vi "BncCore.vi"(8 "error in":errorcluster, 9 "queue error in":errorcluster, 10 "queue in":refnum<queue>, 11 "VISA resource":refnum<visa-resource-name>) -> (0 "error out":errorcluster, 2 "queue out":refnum<queue>)   [LabVIEW 2014]
uses:
  BNC_States.ctl
  SetSystemTypedef.ctl
  Command/Set C-Input.ctl
  Channel.ctl
  Command/Set C-Mode.ctl
  Command/Set C-Output.ctl
  Command/Set C-Enable.ctl
  <instrlib>/BNC/Public/Configure/Configure Sys (To) Mode (Single Shot).vi
  <instrlib>/BNC/Public/Configure/Configure Sys (To) Mode (Normal).vi
  <instrlib>/BNC/Public/Configure/Configure Sys (To) Mode (Duty Cycle).vi
  <instrlib>/BNC/Public/Configure/Configure Sys (To) Mode (Burst).vi
  <instrlib>/BNC/Public/Configure/Configure Chan Mode (Normal).vi
  <instrlib>/BNC/Berkeley Nucleonics 500 Series.lvlib
  <userlib>/Utility/ErrorLog_lib.lvlib
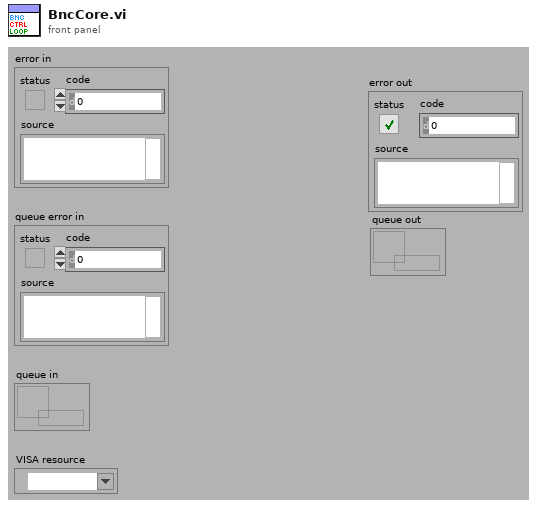
[diagram p1: front panel]
types:
  T1 = typedef "SetSystemTypedef.ctl" = cluster{"Mode":enum16{"Normal", "Single Shot", "Duty Cycle", "Burst"}, "Sys Ext Mode":enum16{"Disabled", "Triggered", "Gated", "Triggered & Gated"}, "Rep.Rate":dbl, "Burst#":i32}
  T2 = enum16{"Disabled", "Pulse Inhibit", "Output Inhibit", "Channel"}
  T3 = typedef "Set C-Input.ctl" = cluster{"Channel":T4, "Sync Source":T4}
  T4 = typedef "Channel.ctl" = i32
  T5 = typedef "Set C-Mode.ctl" = cluster{"Channel":T4, "Delay":dbl, "Width":dbl}
  T6 = typedef "Set C-Output.ctl" = cluster{"Channel":T4, "Polarity":bool}
  T7 = typedef "Set C-Enable.ctl" = cluster{"Channel":T4, "Enable":bool}
  T8 = typedef "BNC_States.ctl" = cluster{"State":enum16{"Initialize", "Set System", "Set C-Input", "Set C-Mode", "Set C-Output", "Set C-Enable", "Manl_Trig", "Run", "Stop", "Query C Number", "Query Status", "Close", "Quit"}, "Para.":variant}
  T9 = enum16{"Initialize", "Set System", "Set C-Input", "Set C-Mode", "Set C-Output", "Set C-Enable", "Manl_Trig", "Run", "Stop", "Query C Number", "Query Status", "Close", "Quit"}
  T10 = enum16{"Normal", "Single Shot", "Duty Cycle", "Burst"}
  T11 = enum16{"Disabled", "Triggered", "Gated", "Triggered & Gated"}
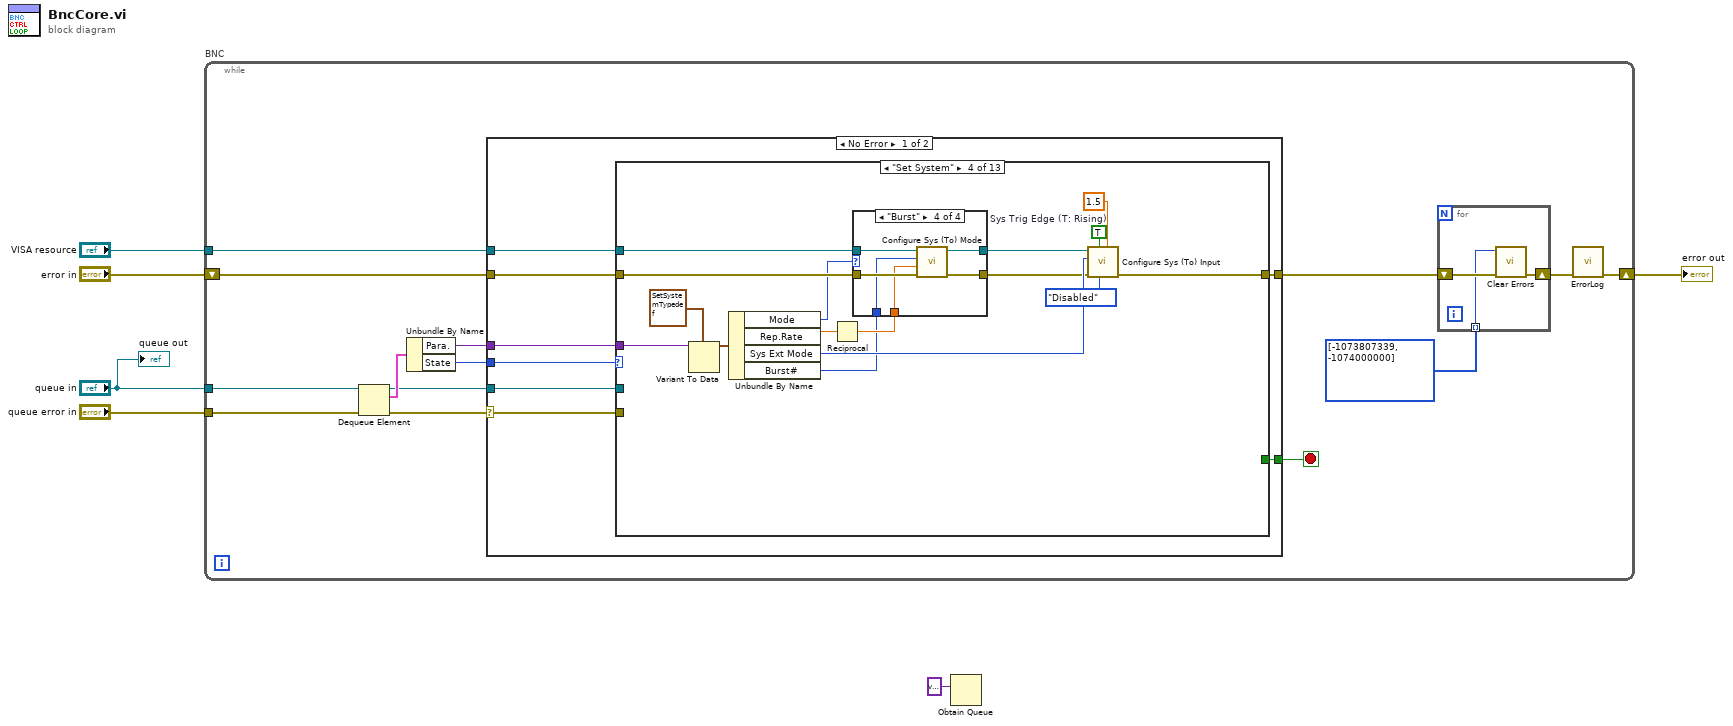
[diagram p0: block diagram]
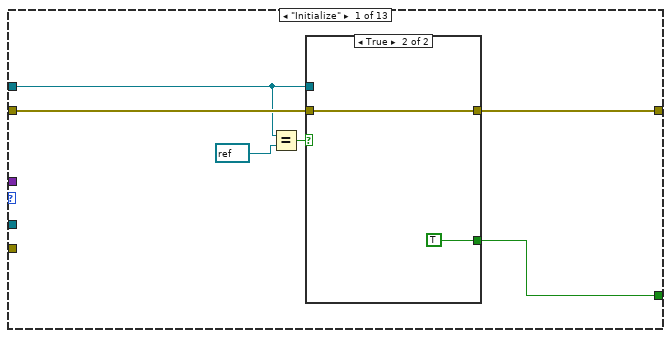
[diagram p2: hidden frame]
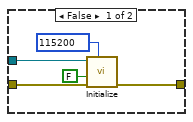
[diagram p3: hidden frame]
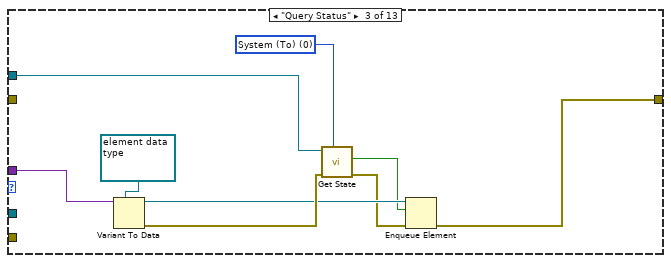
[diagram p5: hidden frame]
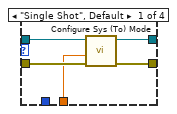
[diagram p6: hidden frame]
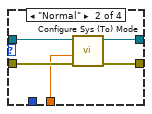
[diagram p7: hidden frame]
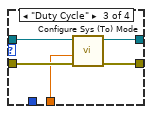
[diagram p8: hidden frame]
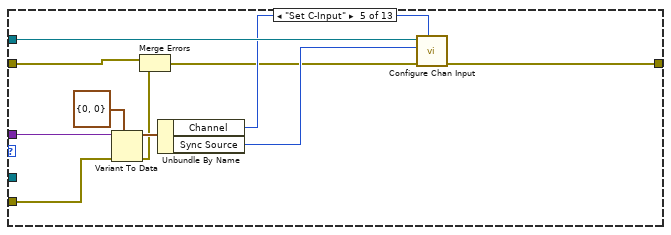
[diagram p9: hidden frame]
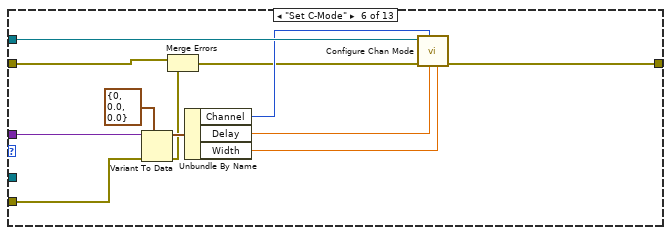
[diagram p10: hidden frame]
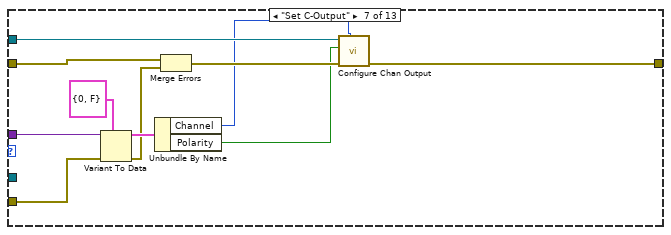
[diagram p11: hidden frame]
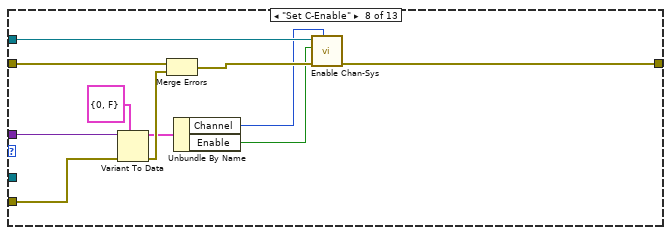
[diagram p12: hidden frame]
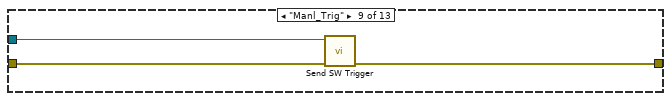
[diagram p13: hidden frame]
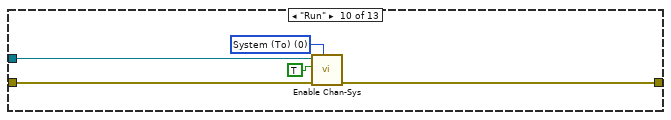
[diagram p14: hidden frame]
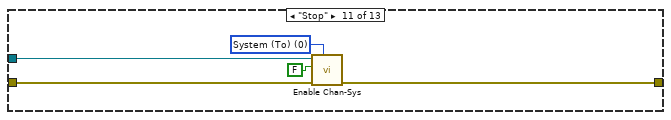
[diagram p15: hidden frame]
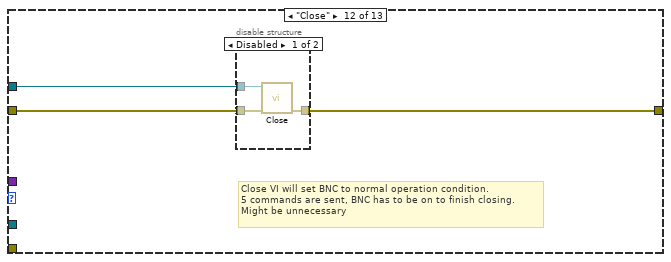
[diagram p16: hidden frame]
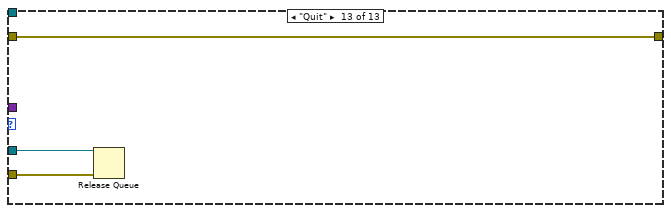
[diagram p18: hidden frame]
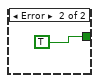
[diagram p19: hidden frame]
diagram:
  n1 = while "BNC" {
    tunnel: "queue in" -> [w20]
    tunnel: "VISA resource" -> [w15]
    shift-right: [w7] -> w2
    shift-left: "error in" -> [w10]
    tunnel: "queue error in" -> [w11]
    stop <- w12 stop-if-true
    n2 = Dequeue Element(queue=w20, error in (no error)=w11) -> (queue out=w16:refnum<queue>, element=w19:T8, error out=w13:errorcluster)  [unwired: 1 in, 1 out]
    n3 = Unbundle By Name(w19) -> ("Para."=w17:variant, "State"=w18:T9)
    n4 = case shown="No Error" w13 {
      selector: w13 -> [w26 _]
      tunnel: w18 -> [w31 _]
      tunnel: w17 -> [w30 _]
      tunnel: w16 -> [w29 _]
      tunnel: w15 -> [w28 _]
      tunnel: w10 -> [w27 _]
      tunnel: [w25 _] -> w14
      tunnel: [w24 TRUE] -> w12
      frame No Error {
        n5 = case shown="\"Set System\"" w31 {
          tunnel: w26 -> [_ _ _ _ w99 w110 w120 w131 _ _ _ _ w158]
          tunnel: w30 -> [_ _ w51 w65 w100 w113 w121 w133 _ _ _ _ _]
          tunnel: w29 -> [_ _ _ _ _ _ _ _ _ _ _ _ w159]
          tunnel: w28 -> [w33 _ w54 w69 w101 w114 w125 w135 w137 w142 w147 w151 _]
          tunnel: w27 -> [w37 w45 _ w70 w92 w103 w117 w136 w139 w143 w148 w152 w157]
          tunnel: [w36 w45 w47 w68 w102 w112 w124 w134 w138 w141 w146 w150 w157] -> w25
          tunnel: [w32 _ _ _ _ _ _ _ _ _ _ _ _] -> w24
          frame "Initialize" {
            n6 = Equal?(x=w33, y=refnum<visa-resource-name> refnum ("VISA resource")) -> (x = y?=w35:bool)
            n7 = case shown="True" w35 {
              tunnel: w33 -> [w42 _]
              tunnel: w37 -> [w41 w44]
              tunnel: [w40 w44] -> w36
              tunnel: [_ TRUE] -> w32
              frame False {
                w38 = u32 115200 items=["4800"=4600, "9600"=9600, "19200"=19200, "38400"=38400, "57600"=57600, "115200"=115200] ("Baud Rate (115200)")
                n8 = call <instrlib>:"Initialize.vi"("Baud Rate (115200)"=w38, "error in (no error)"=w41, "Reset? (T: Yes)"=FALSE, "VISA resource name"=w42) -> ("error out"=w40:errorcluster)  [unwired: 6 in, 1 out]
              }
              frame True {
              }
            }
          }
          frame "Query C Number" {
          }
          frame "Query Status" {
            w53 = 0 items=["System (To)", "Channel A", "Channel B", "Channel C", "Channel D", "Channel E", "Channel F", "Channel G", "Channel H"] ("Channel (1: Chan A)")
            n9 = Variant To Data(type=refnum<queue> refnum ("queue out"), Variant=w51) -> (data=w49:refnum<queue>, error out=w50:errorcluster)  [unwired: 1 in]
            n10 = call <instrlib>:"Get State.vi"("Channel (1: Chan A)"=w53, "error in (no error)"=w50, "VISA resource name"=w54) -> ("error out"=w46:errorcluster, "State"=w48:bool)  [unwired: 6 in, 1 out]
            n11 = Enqueue Element(queue=w49, element=w48, error in (no error)=w46) -> (error out=w47:errorcluster)  [unwired: 1 in, 2 out]
          }
          frame "Set System" {
            w64 = TRUE  # Sys Trig Edge (T: Rising)
            n12 = Variant To Data(type=T1 {"Mode"=enum."Normal", "Sys Ext Mode"=enum."Triggered", "Rep.Rate"=0.0, "Burst#"=1}, Variant=w65) -> (data=w62:T1)  [unwired: 1 in, 1 out]
            n13 = Unbundle By Name(w62) -> ("Mode"=w58:T10, "Rep.Rate"=w60:dbl, "Sys Ext Mode"=w61:T11, "Burst#"=w55:i32)
            n14 = Reciprocal(x=w60) -> (1/x=w59:dbl)
            n15 = case shown="\"Burst\"" w58 {
              tunnel: w70 -> [w75 w80 w85 w91]
              tunnel: w69 -> [w74 w79 w84 w90]
              tunnel: [w73 w78 w83 w89] -> w57
              tunnel: [w72 w77 w82 w88] -> w67
              tunnel: w59 -> [w71 w76 w81 w87]
              tunnel: w55 -> [_ _ _ w86]
              frame "Single Shot", Default {
                n16 = call-poly <instrlib>:"Configure Sys (To) Mode.vi"("error in (no error)"=w75, "Period (100 msec)"=w71, "VISA resource name"=w74) -> ("error out"=w73:errorcluster, "VISA resource name out"=w72:refnum<visa-resource-name>)  [unwired: 7 in]
              }
              frame "Normal" {
                n17 = call-poly <instrlib>:"Configure Sys (To) Mode.vi"("error in (no error)"=w80, "Period (100 msec)"=w76, "VISA resource name"=w79) -> ("error out"=w78:errorcluster, "VISA resource name out"=w77:refnum<visa-resource-name>)  [unwired: 7 in]
              }
              frame "Duty Cycle" {
                n18 = call-poly <instrlib>:"Configure Sys (To) Mode.vi"("error in (no error)"=w85, "Period (100 msec)"=w81, "VISA resource name"=w84) -> ("error out"=w83:errorcluster, "VISA resource name out"=w82:refnum<visa-resource-name>)  [unwired: 7 in]
              }
              frame "Burst" {
                n19 = call-poly <instrlib>:"Configure Sys (To) Mode.vi"("error in (no error)"=w91, "Period (100 msec)"=w87, "Burst # (10)"=w86, "VISA resource name"=w90) -> ("error out"=w89:errorcluster, "VISA resource name out"=w88:refnum<visa-resource-name>)  [unwired: 6 in]
              }
            }
            n20 = call <instrlib>:"Configure Sys (To) Input.vi"("Sys Trig Lev (2.5)"=1.5, "Sys Gate Mode"=T2."Disabled", "Sys Trig Edge (T: Rising)"=w64, "error in (no error)"=w57, "Sys Ext Mode"=w61, "VISA resource name"=w67) -> ("error out"=w68:errorcluster)  [unwired: 4 in, 1 out]
          }
          frame "Set C-Input" {
            n21 = Variant To Data(error in=w99, type=T3 {"Channel"=0, "Sync Source"=0} ("cluster"), Variant=w100) -> (data=w97:T3, error out=w94:errorcluster)
            n22 = Merge Errors(w92, w94) -> (w93:errorcluster)
            n23 = Unbundle By Name(w97) -> ("Channel"=w96:T4, "Sync Source"=w95:T4)
            n24 = call <instrlib>:"Configure Chan Input.vi"("Channel (1:Chan A)"=w96, "error in (no error)"=w93, "Sync Source (0:To)"=w95, "VISA resource name"=w101) -> ("error out"=w102:errorcluster)  [unwired: 6 in, 1 out]
          }
          frame "Set C-Mode" {
            n25 = Variant To Data(error in=w110, type=T5 {"Channel"=0, "Delay"=0.0, "Width"=0.0} ("cluster"), Variant=w113) -> (data=w109:T5, error out=w105:errorcluster)
            n26 = Merge Errors(w103, w105) -> (w104:errorcluster)
            n27 = Unbundle By Name(w109) -> ("Channel"=w108:T4, "Delay"=w107:dbl, "Width"=w106:dbl)
            n28 = call-poly <instrlib>:"Configure Chan Mode.vi"("Width (10 msec)"=w106, "Delay (10 msec)"=w107, "Channel (1:Chan A)"=w108, "error in (no error)"=w104, "VISA resource name"=w114) -> ("error out"=w112:errorcluster)  [unwired: 5 in, 1 out]
          }
          frame "Set C-Output" {
            n29 = Variant To Data(error in=w120, type=T6 {"Channel"=0, "Polarity"=FALSE} ("cluster"), Variant=w121) -> (data=w123:T6, error out=w119:errorcluster)
            n30 = Unbundle By Name(w123) -> ("Channel"=w116:T4, "Polarity"=w115:bool)
            n31 = Merge Errors(w117, w119) -> (w118:errorcluster)
            n32 = call <instrlib>:"Configure Chan Output.vi"("Channel (1:Chan A)"=w116, "error in (no error)"=w118, "Polarity (F:Normal)"=w115, "VISA resource name"=w125) -> ("error out"=w124:errorcluster)  [unwired: 6 in, 1 out]
          }
          frame "Set C-Enable" {
            n33 = Variant To Data(error in=w131, type=T7 {"Channel"=0, "Enable"=FALSE} ("cluster"), Variant=w133) -> (data=w128:T7, error out=w130:errorcluster)
            n34 = Merge Errors(w136, w130) -> (w129:errorcluster)
            n35 = Unbundle By Name(w128) -> ("Channel"=w126:T4, "Enable"=w127:bool)
            n36 = call <instrlib>:"Enable Chan-Sys.vi"("Channel (1:Chan A)"=w126, "error in (no error)"=w129, "State (T:Enabled)"=w127, "VISA resource name"=w135) -> ("error out"=w134:errorcluster)  [unwired: 6 in, 1 out]
          }
          frame "Manl_Trig" {
            n37 = call <instrlib>:"Send SW Trigger.vi"("error in (no error)"=w139, "VISA resource name"=w137) -> ("error out"=w138:errorcluster)  [unwired: 8 in, 1 out]
          }
          frame "Run" {
            w144 = 0 items=["System (To)", "Channel A", "Channel B", "Channel C", "Channel D", "Channel E", "Channel F", "Channel G", "Channel H"] ("Channel (1:Chan A)")
            n38 = call <instrlib>:"Enable Chan-Sys.vi"("Channel (1:Chan A)"=w144, "error in (no error)"=w143, "State (T:Enabled)"=TRUE, "VISA resource name"=w142) -> ("error out"=w141:errorcluster)  [unwired: 6 in, 1 out]
          }
          frame "Stop" {
            w149 = 0 items=["System (To)", "Channel A", "Channel B", "Channel C", "Channel D", "Channel E", "Channel F", "Channel G", "Channel H"] ("Channel (1:Chan A)")
            n39 = call <instrlib>:"Enable Chan-Sys.vi"("Channel (1:Chan A)"=w149, "error in (no error)"=w148, "State (T:Enabled)"=FALSE, "VISA resource name"=w147) -> ("error out"=w146:errorcluster)  [unwired: 6 in, 1 out]
          }
          frame "Close" {
            # "Close VI will set BNC to normal operation condition.\n5 commands are sent, BNC has to be on to finish closing.\nMight be unnecessary"
            n40 = disable-structure shown="Disabled" {
              disable-tunnel: w152 -> [w155 w156]
              disable-tunnel: w151 -> [w154 _]
              disable-tunnel: [w153 w156] -> w150
              frame Disabled {
                n41 = call <instrlib>:"Close.vi"("error in (no error)"=w155, "VISA resource name"=w154) -> ("error out"=w153:errorcluster)  [unwired: 9 in]
              }
              frame Enabled {
              }
            }
          }
          frame "Quit" {
            n42 = Release Queue(queue=w159, error in (no error)=w158) -> ()  [unwired: 1 in, 3 out]
          }
        }
      }
      frame Error {
      }
    }
    n43 = for {
      tunnel: i32[] [-1073807339, -1074000000] -> [w21] mode=indexing
      shift-right: [w22] -> w9
      shift-left: w14 -> [w23]
      n44 = call <vilib>:"Clear Errors.vi"("error in (no error)"=w23, "specific error code to clear (0: all)"=w21) -> ("error out"=w22:errorcluster)  [unwired: 4 in, 1 out]
    }
    n45 = call <userlib>:"ErrorLog.vi"("error in (no error)"=w9) -> ("error out"=w7:errorcluster)  [unwired: 10 in]
  }
  "error out" <- w2
  n46 = Obtain Queue(element data type=variant) -> ()  [unwired: 4 in, 3 out]
  "queue out" <- "queue in"
